vi "get tag by name.vi"(8 "error in":errorcluster, 10 "tag":string, 11 "tag collection in":refnum<class "tag collection.lvclass">) -> (0 "error out":errorcluster, 1 "located tag":refnum<class "tag descriptor.lvclass">, 3 "tag collection out":refnum<class "tag collection.lvclass">)   [LabVIEW 2013, in "tag collection.lvclass"]
uses:
  tag collection.lvclass
  tag/tag descriptor.lvclass
  tag collection.lvclass/tag collection.ctl
  tag/tag descriptor.lvclass/tag descriptor.ctl
  tag/read tag name.vi
  tag bus.lvlib
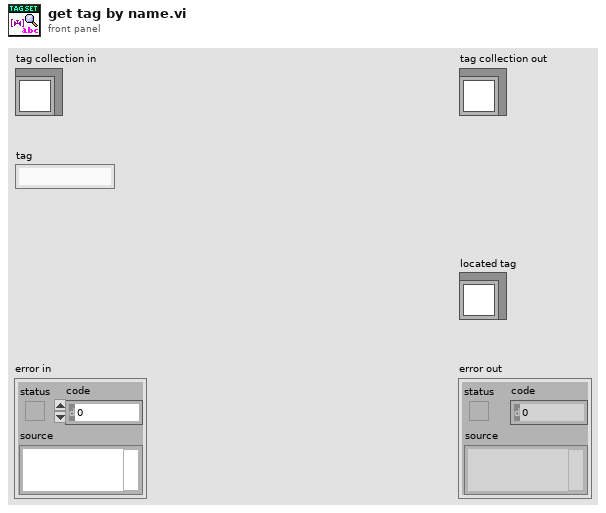
[diagram p1: front panel]
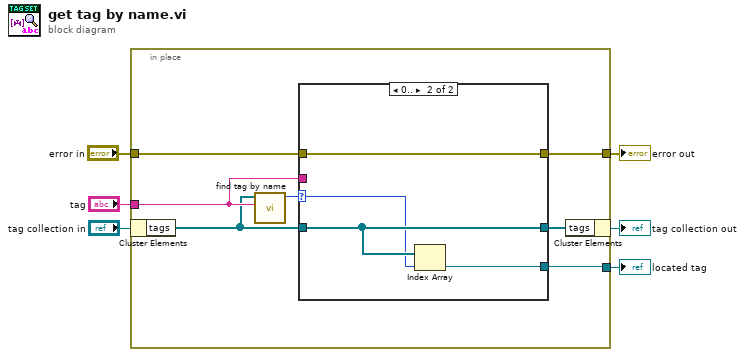
[diagram p0: block diagram]
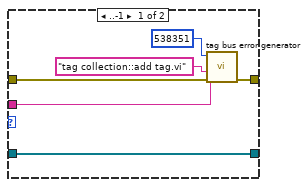
[diagram p2: hidden frame]
diagram:
  n1 = in-place {
    in-place-border: "error in" -> [w12]
    in-place-border: [w13] -> w3
    in-place-border: "tag" -> [w9]
    in-place-border: [w7] -> w1
    n2 = in-place-cluster #1("tag collection in") -> ("tags"=w8:refnum<class "tag descriptor.lvclass">[])
    n3 = call "find tag by name.vi"("name"=w9, "tags in"=w8) -> ("index"=w10:i32)  [unwired: 9 in]
    n4 = case shown="0.." w10 {
      selector: w10 -> [_ w20]
      tunnel: [w17 w23] -> w13
      tunnel: w12 -> [w18 w23]
      tunnel: w8 -> [w19 w21]
      tunnel: [w19 w21] -> w11
      tunnel: w9 -> [w14 _]
      tunnel: [_ w22] -> w7
      frame ..-1 {
        n5 = call "tag bus error generator.vi"("error in"=w18, "source"="tag collection::add tag.vi", "append error message"=w14, "error code (0)"=538351) -> ("error out"=w17:errorcluster)  [unwired: 5 in]
      }
      frame 0.. {
        n6 = Index Array(array=w21, index=w20) -> (element=w22:refnum<class "tag descriptor.lvclass">)
      }
    }
    n7 = in-place-cluster #1("tags"=w11) -> (→"tag collection out":refnum<class "tag collection.lvclass">)
  }
  "error out" <- w3
  "located tag" <- w1
